vi "Get Measurement Details.vi"(8 "error in":errorcluster) -> (0 "error out":errorcluster, 2 "service class":string, 3 "measurement details":T1)   [LabVIEW 2021, in "adc_fullScaleError.lvlib"]
uses:
  adc_fullScaleError.lvlib
  <vilib>/MeasurementLink/MeasurementLink Measurement Server Internal/RPC Messages/ni_measurementlink_measurement_v1_MeasurementDetails.ctl
  <vilib>/MeasurementLink/MeasurementLink Measurement Server Internal/MeasurementLink Measurement Server Internal.lvlib
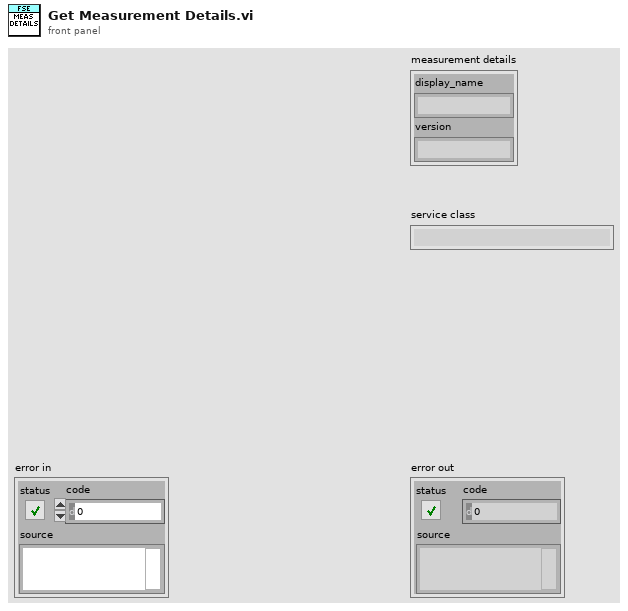
[diagram p1: front panel]
types:
  T1 = typedef "MeasurementLink Measurement Server Internal.lvlib/ni_measurementlink_measurement_v1_MeasurementDetails.ctl" = cluster{"display_name":string, "version":string}
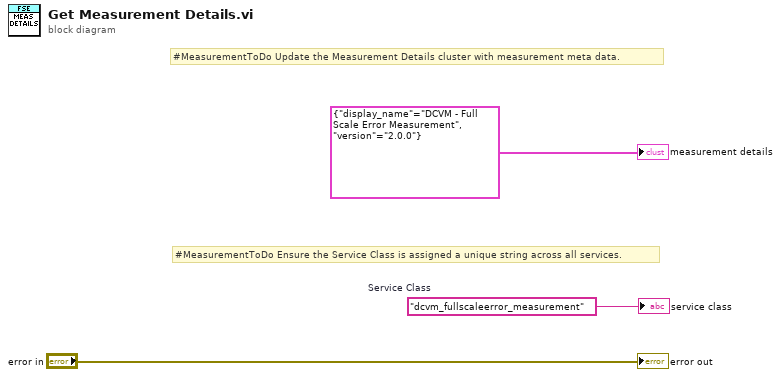
[diagram p0: block diagram]
diagram:
  w2 = "dcvm_fullscaleerror_measurement"  # Service Class
  # "#MeasurementToDo Ensure the Service Class is assigned a unique string across all services."
  # "#MeasurementToDo Update the Measurement Details cluster with measurement meta data."
  "error out" <- "error in"
  "measurement details" <- T1 {"display_name"="DCVM - Full Scale Error Measurement", "version"="2.0.0"} ("Measurement Details")
  "service class" <- w2
